vi "Single-Element Write to file.vi"(7 "refnum":refnum<file>, 10 "sorted 2D array":dbl[](array[numeric])) -> (0 "error out":errorcluster, 3 "resulting string":string)   [LabVIEW 2020]
panel:
  out "Byte Stream File out":refnum<file>
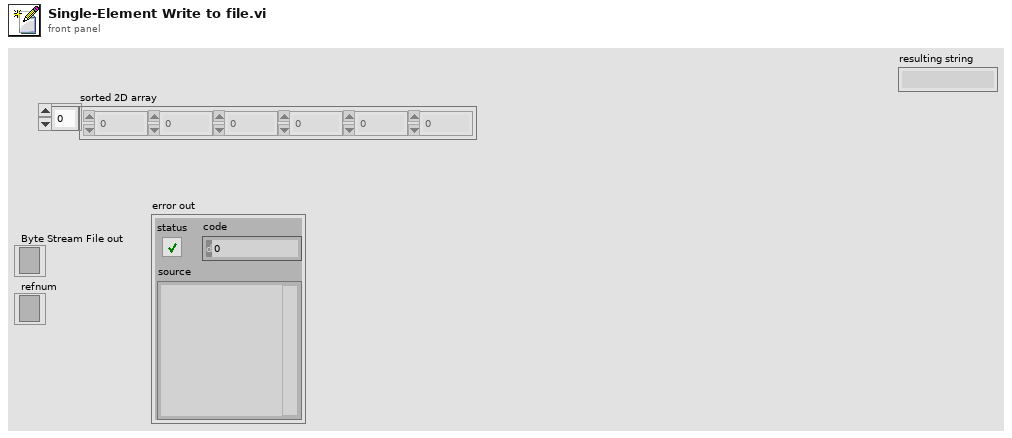
[diagram p1: front panel]
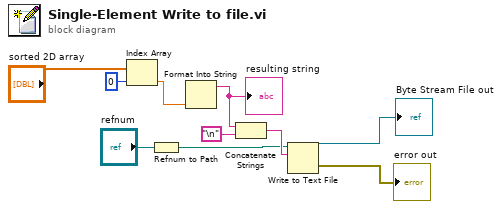
[diagram p0: block diagram]
diagram:
  n1 = Index Array(array="sorted 2D array", index=0) -> (element=w10:dbl)
  n2 = Refnum to Path(1:"refnum") -> (0:w2:path)
  n3 = Format Into String(w10) -> (resulting string=w8:string)  [unwired: 3 in, 1 out]
  "resulting string" <- w8
  n4 = Concatenate Strings(w8, "\n") -> (w9:string)
  n5 = Write to Text File(file (use dialog)=w2, text=w9) -> (refnum out=→"Byte Stream File out":refnum<file>, error out=→"error out":errorcluster)  [unwired: 2 in, 1 out]
